vi "N10_Frisbee_Shooter.vi"() -> ()   [LabVIEW 2023]
panel:
  out "Armed":bool
  out "Shoot":bool
  in  "Command Shoot":bool
  in  "Shooter Angle":dbl(slide) scale=0.0..75.0
  # "A slider controls the angle of a frisbee shooter\n\nRequirements\n- When the angle of the frisbee shooter is less than 40 degrees disarm the shooter.\n- When the angle of the frisbee shooter is greater than or equal to than 40 degrees arm  the shooter.\n- When the shoot button is pressed and the the shooter is armed, shoot the frisbee."
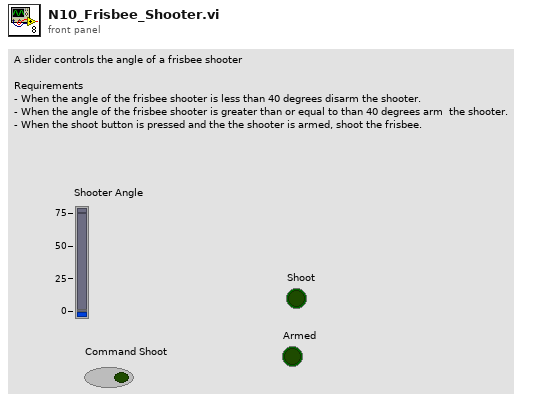
[diagram p1: front panel]
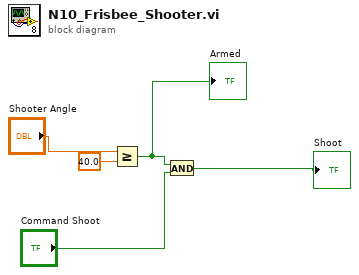
[diagram p0: block diagram]
diagram:
  n1 = Greater Or Equal?(x="Shooter Angle", y=40.0) -> (x >= y?=w1:bool)
  "Armed" <- w1
  n2 = And(x=w1, y="Command Shoot") -> (x .and. y?=→"Shoot":bool)
